vi "UI_Set Focus.vi"(8 "Error":errorcluster, 9 "Focus Select":T1, 11 "Ref String  Array":refnum<vi>[](array[refnum])) -> (0 "Error Out":errorcluster)   [LabVIEW 2009]
doc: "Sets a string control as focus based on selection"
uses:
  Controls/Enum/ENUM_Set Focus Select.ctl
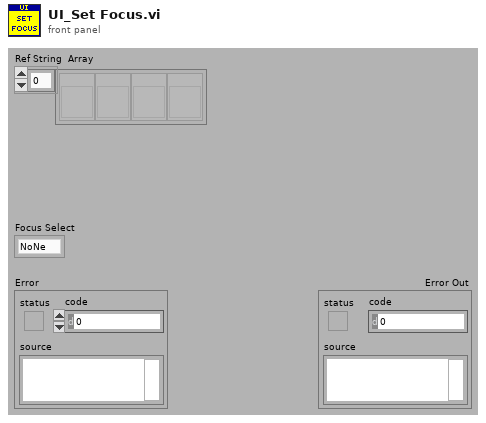
[diagram p1: front panel]
types:
  T1 = typedef "ENUM_Set Focus Select.ctl" = enum16{"NoNe", "Header", "Line 1", "Line 2", "Line 3", "Line 4", "Next", "Back"}
  T2 = cluster{"Selection Start":u32, "Selection End":u32}
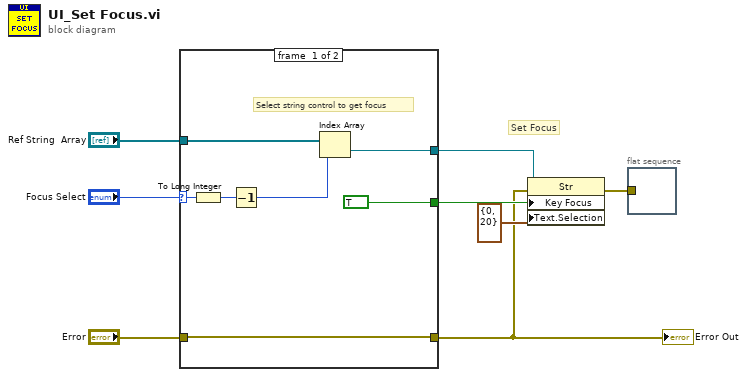
[diagram p0: block diagram]
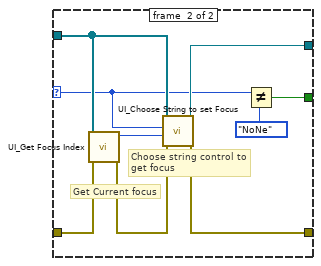
[diagram p2: hidden frame]
diagram:
  # "Set Focus"
  n1 = case shown="\"NoNe\", \"Next\", \"Back\"" "Focus Select" {
    selector: "Focus Select" -> [w13 w18]
    tunnel: "Ref String  Array" -> [w15 w22]
    tunnel: [w14 w19] -> w7
    tunnel: [TRUE ("Key Focus") w16] -> w5
    tunnel: "Error" -> [w10 w24]
    tunnel: [w10 w20] -> w2
    frame #0 {
      # "Select string control to get focus"
      n2 = To Long Integer(number=w13) -> (32bit integer=w9:i32)
      n3 = Decrement(x=w9) -> (x-1=w12:i32)
      n4 = Index Array(array=w15, index=w12) -> (element=w14:refnum<vi>)
    }
    frame #1 {
      # "Choose string control to \nget focus"
      # "Get Current focus"
      n5 = call "UI_Get Focus Index.vi"("Error"=w24, "Ref String  Array"=w22) -> ("Error Out"=w21:errorcluster, "Focus Index Out"=w23:i32)  [unwired: 8 in]
      n6 = call "UI_Choose String to set Focus.vi"("Error"=w21, "Current Index"=w23, "Focus Select"=w18, "Ref String  Array"=w22) -> ("Error Out"=w20:errorcluster, "String Ref Out"=w19:refnum<vi>)  [unwired: 5 in, 1 out]
      n7 = Not Equal?(x=w18, y=ENUM_Set_Focus_Select."NoNe") -> (x != y?=w16:bool)
    }
  }
  "Error Out" <- w2
  n8 = property class="Str"(reference=w7, error in=w2, "Key Focus"=w5, "Text.Selection"=T2 {"Selection Start"=0, "Selection End"=20}) -> (error out=w1:errorcluster)  [unwired: 1 out]
  n9 = flat-sequence {
    tunnel: w1 -> [_]
    frame #0 {
    }
  }
